vi "To Serial Form.vi"(6 "Serial Version":T1, 10 "Serializer in":refnum<class "Serializer.lvclass">, 11 "CRDS Data in":refnum<class "CRDS Data.lvclass">) -> (0 "error out":errorcluster, 2 "Serializer out":refnum<class "Serializer.lvclass">, 3 "CRDS Data out":refnum<class "CRDS Data.lvclass">)   [LabVIEW 2014, in "CRDS Data.lvclass"]
uses:
  CRDS Data.lvclass
  <vilib>/NI/AQ Character Lineator/Serializer/Serializer.lvclass
  <vilib>/NI/AQ Character Lineator/Serialization Common/Serial Version.ctl
  Cell/CRDS Cell Data.lvclass
  CRDS Data.lvclass/CRDS Data.ctl
  <vilib>/NI/AQ Character Lineator/Serializable/Insert Single.vi
  <vilib>/NI/AQ Character Lineator/Serializer/Insert Single.vi
  <vilib>/NI/AQ Character Lineator/Serializer/Read Include Default Values.vi
  Data/Data.lvclass
  <vilib>/NI/AQ Character Lineator/Serializable/Serializable.lvclass
  <vilib>/NI/AQ Character Lineator/Serialization Common/Serialization Common.lvlib
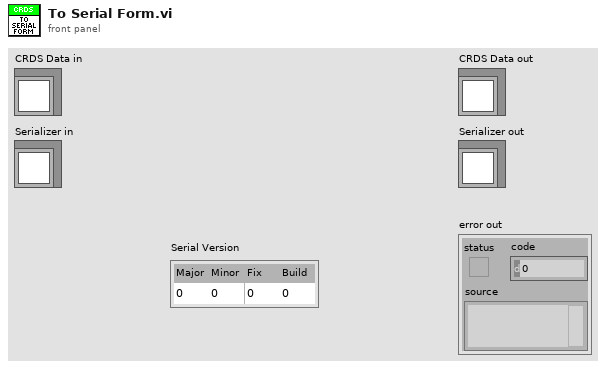
[diagram p1: front panel]
types:
  T1 = typedef "Serialization Common.lvlib/Serial Version.ctl" = cluster{"Major":u16, "Minor":u16, "Fix":u16, "Build":u16}
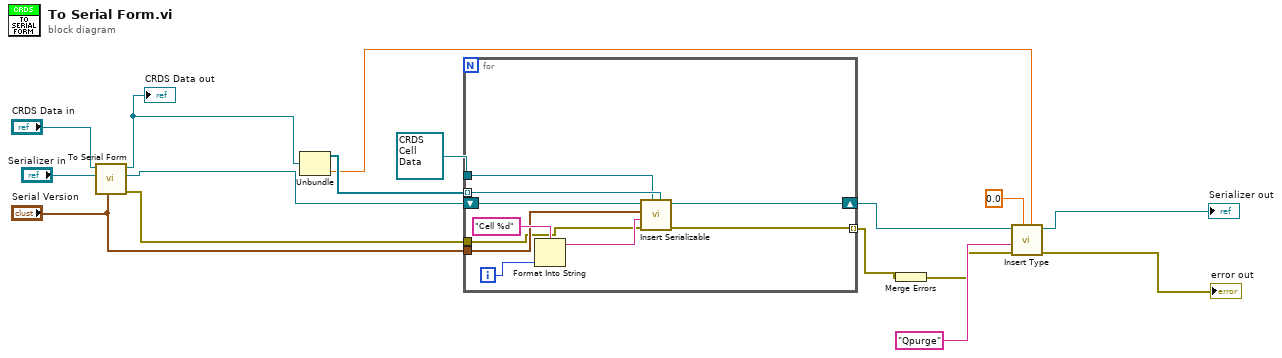
[diagram p0: block diagram]
diagram:
  n1 = call-parent "To Serial Form.vi"("Serial Version"="Serial Version", "Serializer in"="Serializer in", "Data in"="CRDS Data in") -> ("error out"=w10:errorcluster, "Serializer out"=w2:refnum<class "Serializer.lvclass">, "Data out"=w14:refnum<class "CRDS Data.lvclass">)  [unwired: 6 in]
  "CRDS Data out" <- w14
  n2 = Unbundle(w14) -> (w13:refnum<class "CRDS Cell Data.lvclass">[], w8:sgl)  [unwired: 1 out]
  n3 = for {
    tunnel: w13 -> [w26] mode=indexing
    tunnel: refnum<class "CRDS Cell Data.lvclass"> refnum ("CRDS Cell") -> [w25]
    shift-right: [w21] -> w9
    shift-left: w2 -> [w20]
    tunnel: "Serial Version" -> [w19]
    tunnel: w10 -> [w18]
    tunnel: [w17] -> w5 mode=indexing
    i -> [w24]
    n4 = Format Into String(format string="Cell %d", w24) -> (resulting string=w22:string)  [unwired: 2 in, 1 out]
    n5 = call <vilib>:"Insert Serializable.vi"("Serializable"=w26, "Default Value"=w25, "error in (no error)"=w18, "Name"=w22, "Serial Version"=w19, "Serializer in"=w20) -> ("error out"=w17:errorcluster, "Serializer out"=w21:refnum<class "Serializer.lvclass">)  [unwired: 4 in]
  }
  n6 = Merge Errors(w5) -> (w4:errorcluster)
  n7 = call-poly <vilib>:"Insert Type.vi"("Double"=w8, "Default Value"=sgl 0.0, "error in (no error)"=w4, "Name"="Qpurge", "Serializer in"=w9) -> ("error out"=→"error out":errorcluster, "Serializer out"=→"Serializer out":refnum<class "Serializer.lvclass">)  [unwired: 5 in]
